vi "closeAnalysis.vi"(8 "error in (no error)":errorcluster, 11 "ImageStreamViewer in":refnum<class "ImageStreamViewer.lvclass">) -> (0 "error out":errorcluster, 3 "ImageStreamViewer out":refnum<class "ImageStreamViewer.lvclass">)   [LabVIEW 2009, in "Views.lvlib" / "Camera.lvlib" / "ImageStreamViewer.lvclass"]
doc: "This vi sends \"closeEvents\" to the analysis runner. It waits until the vi reference has been disposed of by labview."
uses:
  ImageStreamViewer.lvclass
  ImageStreamViewer.lvclass/ImageStreamViewer.ctl
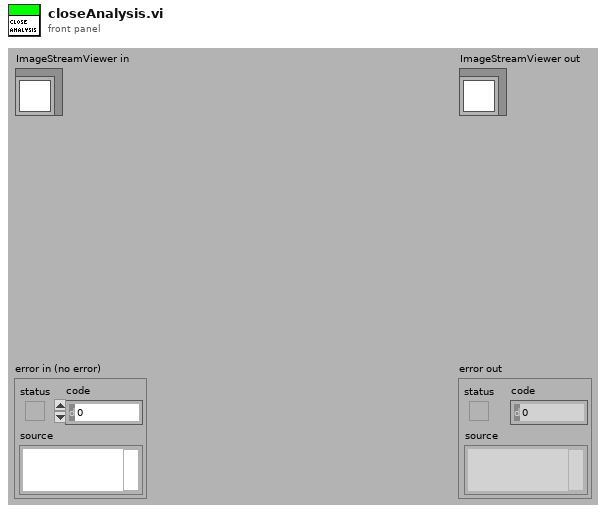
[diagram p1: front panel]
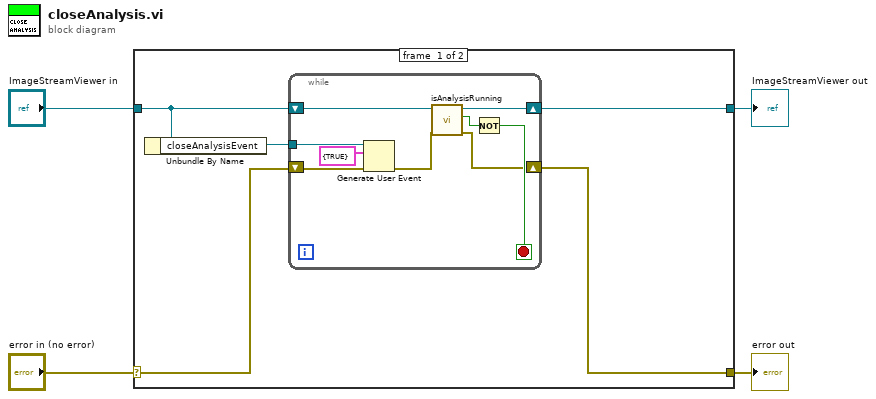
[diagram p0: block diagram]
diagram:
  n1 = case shown="No Error" "error in (no error)" {
    selector: "error in (no error)" -> [w8 w20]
    tunnel: [w5 w20] -> w3
    tunnel: [w6 w19] -> w1
    tunnel: "ImageStreamViewer in" -> [w7 w19]
    frame #0 {
      n2 = Unbundle By Name(w7) -> ("closeAnalysisEvent"=w9:refnum<user-event>)
      n3 = while {
        tunnel: w9 -> [w18]
        shift-right: [w10] -> w5
        shift-left: w8 -> [w15]
        shift-right: [w13] -> w6
        shift-left: w7 -> [w14]
        stop <- w11 stop-if-true
        n4 = Generate User Event(user event=w18, event data cluster=cluster{bool} {TRUE} ("event data"), error in=w15) -> (error out=w17:errorcluster)  [unwired: 1 out]
        n5 = call "isAnalysisRunning.vi"("error in (no error)"=w17, "ImageStreamViewer in"=w14) -> ("error out"=w10:errorcluster, "running?"=w12:bool, "ImageStreamViewer out"=w13:refnum<class "ImageStreamViewer.lvclass">)  [unwired: 7 in]
        n6 = Not(x=w12) -> (.not. x?=w11:bool)
      }
    }
    frame #1 {
    }
  }
  "error out" <- w3
  "ImageStreamViewer out" <- w1
